vi "Drag Label.vi"(0 "FSM.Edge In":refnum<class "FSM.Edge.lvclass">, 9 "delta":T1) -> (4 "FSM.Edge Out":refnum<class "FSM.Edge.lvclass">)   [LabVIEW 2020, in "FSM.Edge.lvclass"]
uses:
  FSM.Edge.lvclass
  <vilib>/Utility/miscctls.llb/LVPoint32TypeDef.ctl
  FSM.Edge.lvclass/FSM.Edge.ctl
  FSM.Label/FSM.Label.lvclass
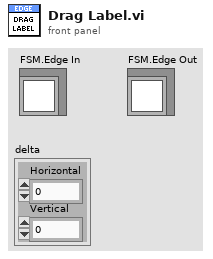
[diagram p1: front panel]
types:
  T1 = typedef "LVPoint32TypeDef.ctl" = cluster{"Horizontal":i32, "Vertical":i32}
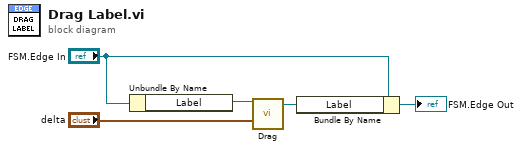
[diagram p0: block diagram]
diagram:
  n1 = Unbundle By Name("FSM.Edge In") -> ("Label"=w5:refnum<class "FSM.Label.lvclass">)
  n2 = call "Drag.vi"("FSM.Label In"=w5, "delta"="delta") -> ("FSM.Label Out"=w3:refnum<class "FSM.Label.lvclass">)  [unwired: 13 in]
  n3 = Bundle By Name(cluster="FSM.Edge In", "Label"=w3) -> (→"FSM.Edge Out":refnum<class "FSM.Edge.lvclass">)
